vi "Rnadom.vi"() -> ()   [LabVIEW 2024]
panel:
  out "Array":dbl[](array[numeric])
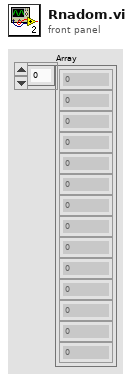
[diagram p1: front panel]
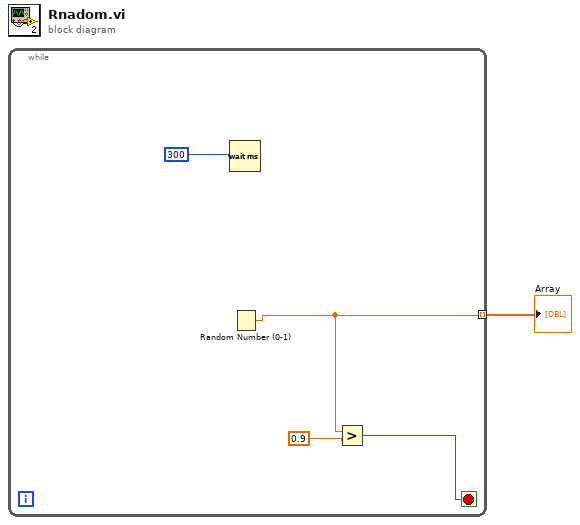
[diagram p0: block diagram]
diagram:
  n1 = while {
    tunnel: [w3] -> w1 mode=indexing
    stop <- w2 stop-if-true
    n2 = Wait (ms)(milliseconds to wait=u32 300) -> ()  [unwired: 1 out]
    n3 = Random Number (0-1)() -> (number: 0 to 1=w3:dbl)
    n4 = Greater?(x=w3, y=0.9) -> (0:w2:bool)
  }
  "Array" <- w1
